vi "PCinfo_Win7.vi"(10 "DLL基路径":path) -> (2 "PC验证结果":bool)   [LabVIEW 2010]
uses:
  PCinfoWin7.dll
panel:
  out "DLL基路径显示":path
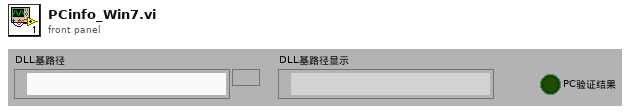
[diagram p1: front panel]
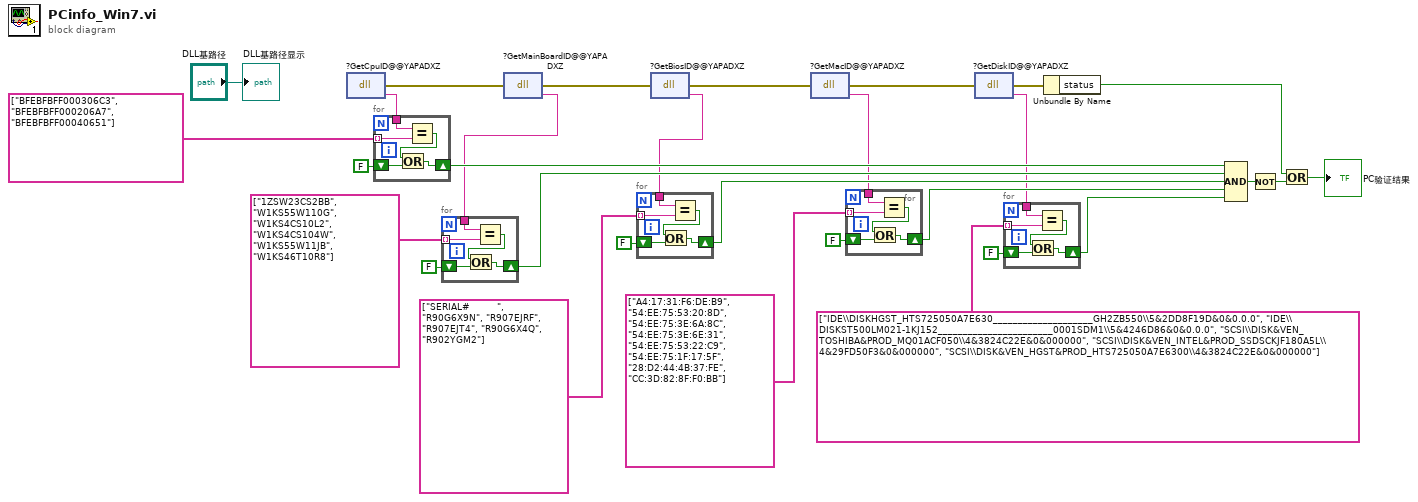
[diagram p0: block diagram]
diagram:
  n1 = dll-call lib="L:/DR-HB型数字化反应性仪工程机_TXT_MB/PCinfoWin7.dll" fn="?GetCpuID@@YAPADXZ" label="CPU（必须首先调用）"() -> (error out=w30:errorcluster, "返回类型"=w26:string)  [unwired: 3 in, 1 out]
  n2 = for {
    tunnel: w26 -> [w35]
    tunnel: string[] ["BFEBFBFF000306C3", "BFEBFBFF000206A7", "BFEBFBFF00040651"] ("添加的数组") -> [w34] mode=indexing
    shift-right: [w33] -> w21
    shift-left: FALSE -> [w32]
    n3 = Equal?(x=w35, y=w34) -> (x = y?=w31:bool)
    n4 = Or(x=w31, y=w32) -> (x .or. y?=w33:bool)
  }
  n5 = dll-call lib="L:/DR-HB型数字化反应性仪工程机_TXT_MB/PCinfoWin7.dll" fn="?GetMainBoardID@@YAPADXZ" label="MainBoard"(error in=w30) -> (error out=w29:errorcluster, "返回类型"=w19:string)  [unwired: 2 in, 1 out]
  n6 = for {
    tunnel: w19 -> [w40]
    tunnel: string[] ["1ZSW23CS2BB", "W1KS55W110G", "W1KS4CS10L2", "W1KS4CS104W", "W1KS55W11JB", "W1KS46T10R8"] ("添加的数组") -> [w39] mode=indexing
    shift-right: [w38] -> w17
    shift-left: FALSE -> [w37]
    n7 = Equal?(x=w40, y=w39) -> (x = y?=w36:bool)
    n8 = Or(x=w36, y=w37) -> (x .or. y?=w38:bool)
  }
  n9 = dll-call lib="L:/DR-HB型数字化反应性仪工程机_TXT_MB/PCinfoWin7.dll" fn="?GetBiosID@@YAPADXZ" label="BIOS"(error in=w29) -> (error out=w28:errorcluster, "返回类型"=w15:string)  [unwired: 2 in, 1 out]
  n10 = for {
    tunnel: w15 -> [w45]
    tunnel: string[] ["SERIAL#         ", "R90G6X9N", "R907EJRF", "R907EJT4", "R90G6X4Q", "R902YGM2"] ("添加的数组") -> [w44] mode=indexing
    shift-right: [w43] -> w13
    shift-left: FALSE -> [w42]
    n11 = Equal?(x=w45, y=w44) -> (x = y?=w41:bool)
    n12 = Or(x=w41, y=w42) -> (x .or. y?=w43:bool)
  }
  n13 = dll-call lib="L:/DR-HB型数字化反应性仪工程机_TXT_MB/PCinfoWin7.dll" fn="?GetMacID@@YAPADXZ" label="First MAC"(error in=w28) -> (error out=w27:errorcluster, "返回类型"=w11:string)  [unwired: 2 in, 1 out]
  n14 = for {
    tunnel: w11 -> [w50]
    tunnel: string[] ["A4:17:31:F6:DE:B9", "54:EE:75:53:20:8D", "54:EE:75:3E:6A:8C", "54:EE:75:3E:6E:31", "54:EE:75:53:22:C9", "54:EE:75:1F:17:5F", "28:D2:44:4B:37:FE", "CC:3D:82:8F:F0:BB"] ("添加的数组") -> [w49] mode=indexing
    shift-right: [w48] -> w10
    shift-left: FALSE -> [w47]
    n15 = Equal?(x=w50, y=w49) -> (x = y?=w46:bool)
    n16 = Or(x=w46, y=w47) -> (x .or. y?=w48:bool)
  }
  n17 = dll-call lib="L:/DR-HB型数字化反应性仪工程机_TXT_MB/PCinfoWin7.dll" fn="?GetDiskID@@YAPADXZ" label="First Disk"(error in=w27) -> (error out=w24:errorcluster, "返回类型"=w7:string)  [unwired: 2 in, 1 out]
  n18 = for {
    tunnel: w7 -> [w55]
    tunnel: string[] ["IDE\\DISKHGST_HTS725050A7E630____________________GH2ZB550\\5&2DD8F19D&0&0.0.0", "IDE\\DISKST500LM021-1KJ152_______________________0001SDM1\\5&4246D86&0&0.0.0", "SCSI\\DISK&VEN_TOSHIBA&PROD_MQ01ACF050\\4&3824C22E&0&000000", "SCSI\\DISK&VEN_INTEL&PROD_SSDSCKJF180A5L\\4&29FD50F3&0&000000", "SCSI\\DISK&VEN_HGST&PROD_HTS725050A7E6300\\4&3824C22E&0&000000"] ("添加的数组") -> [w54] mode=indexing
    shift-right: [w53] -> w6
    shift-left: FALSE -> [w52]
    n19 = Equal?(x=w55, y=w54) -> (x = y?=w51:bool)
    n20 = Or(x=w51, y=w52) -> (x .or. y?=w53:bool)
  }
  n21 = Unbundle By Name(w24) -> ("status"=w1:bool)
  n22 = Compound Arithmetic op=AND(w21, w17, w13, w10, w6) -> (w4:bool)
  n23 = Not(x=w4) -> (.not. x?=w3:bool)
  n24 = Or(x=w1, y=w3) -> (x .or. y?=→"PC验证结果":bool)
  "DLL基路径显示" <- "DLL基路径"
